vi "Search 2D Array (String).vi"(10 "Element":string, 11 "Array":string[][](array[string])) -> (3 "Locations":i32[][](array[numeric]))   [LabVIEW 2020]
uses:
  Search 2D Array (Bool).vi
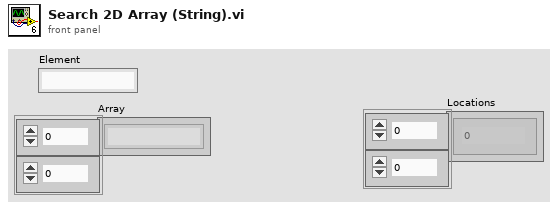
[diagram p1: front panel]
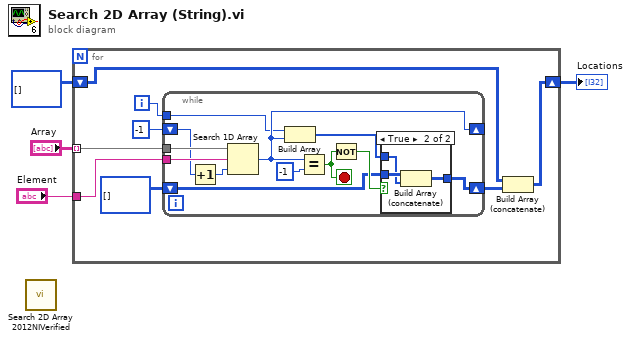
[diagram p0: block diagram]
diagram:
  n1 = call-poly "Search 2D Array 2012NIVerified.vi"() -> ()  [unwired: 11 in, 1 out]
  n2 = for {
    tunnel: "Array" -> [w12] mode=indexing
    tunnel: "Element" -> [w11]
    shift-right: [w6] -> w2
    shift-left: i32[][] [] -> [w7]
    i -> [w10]
    n3 = while {
      tunnel: w12 -> [w24]
      tunnel: w11 -> [w23]
      shift-right: [w20] -> _
      shift-left: -1 ("index of element") -> [w22]
      tunnel: w10 -> [w19]
      shift-right: [w13] -> w9
      shift-left: i32[][] [] ("Array 2") -> [w14]
      stop <- w16 stop-if-true
      n4 = Increment(x=w22) -> (x+1=w17:i32)
      n5 = Search 1D Array(1D array=w24, element=w23, start index (0)=w17) -> (index of element=w20:i32)
      n6 = Build Array(w19, w20) -> (w18:i32[])
      n7 = Equal?(x=w20, y=-1) -> (x = y?=w16:bool)
      n8 = Not(x=w16) -> (.not. x?=w15:bool)
      n9 = case shown="True" w15 {
        tunnel: w14 -> [w25 w27]
        tunnel: w18 -> [_ w26]
        tunnel: [w25 w28] -> w13
        frame False {
        }
        frame True {
          n10 = Build Array (concatenate)(w27, w26) -> (w28:i32[][])
        }
      }
    }
    n11 = Build Array (concatenate)(w7, w9) -> (w6:i32[][])
  }
  "Locations" <- w2
